vi "Dashboard Main.vi"() -> (0 "Camera Image":T3(plugin-control))   [LabVIEW 2011]
uses:
  <vilib>/Rock Robotics/WPI/Camera/WPI_CameraImageSize.ctl
  <vilib>/Rock Robotics/WPI/DriverStation/WPI_DriverStationDigitalData.ctl
  <vilib>/Utility/inputDevices.llb/keyboardAcquire.vi
  <vilib>/Utility/inputDevices.llb/closeKeyboard.vi
panel:
  out "UP":bool
  out "LEFT":bool
  out "RIGHT":bool
  out "DOWN":bool
  out "SPACE":bool
  out "X":dbl
  out "Y":dbl
  out "Target Info":T1(array[cluster])
  in  "Viewer":T2(tab)
  in  "Video Enable":bool=TRUE
  out "Processed Image":T3(plugin-control)
  in  "Range":cluster{"Lower value":sgl, "Upper value":sgl}={"Lower value"=234.67392, "Upper value"=255.0} {"Lower value" scale=0.0..255.0; "Upper value" scale=0.0..255.0}
  in  "Image Size":T4
  in  "1":bool
  in  "2":bool
  in  "3":bool
  in  "4":bool
  out "Selected Target Info":T5
  out "Buttons 1":cluster{"1":bool, "2":bool, "3":bool}
  out "Kinect 1":cluster{"X":dbl, "Y":dbl, "Z":dbl} {"X" scale=1.0..-1.0; "Y" scale=1.0..-1.0; "Z" scale=1.0..-1.0}
  out "Buttons 2":cluster{"1":bool, "2":bool, "3":bool}
  out "Kinect 2":cluster{"X":dbl, "Y":dbl, "Z":dbl} {"X" scale=1.0..-1.0; "Y" scale=1.0..-1.0; "Z" scale=1.0..-1.0}
  out "Version":string
  out "Skeleton Picture":picture
  out "Players":i8
  out "Original Image":T3(plugin-control)
  out "Latched Cordinates":i32[](array[numeric])
  out "?":i32[](array[numeric])
  out "Numeric 2":dbl
  out "Numeric":dbl
  out "distance to basket":dbl
  out "rotation angle":dbl
  in  "Basket Number":i32
  out "Dashboard Datatype Warning":string="Warning: The Dashboard Datatype used by the robot project and this dashboard do not match.\nSee diagram for more details."
  # "1"
  # "2"
  # "3"
  # "4"
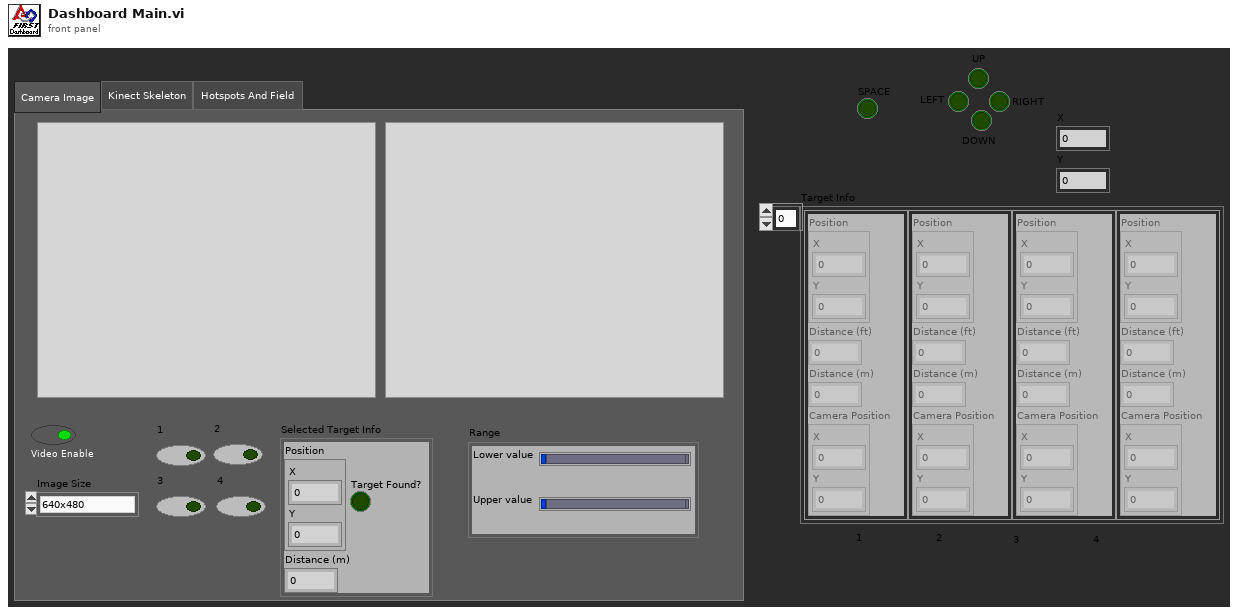
[diagram p1: front panel]
types:
  T1 = cluster{"Position":cluster{"X":dbl, "Y":dbl}, "Distance (ft)":dbl, "Distance (m)":dbl, "Camera Position":cluster{"X":dbl, "Y":dbl}}[]
  T2 = enum32{"Camera Image", "Kinect Skeleton", "Hotspots And Field "}
  T3 = typedef "IMAQ Image.ctl" = refnum<image>
  T4 = typedef "WPI_CameraImageSize.ctl" = enum16{"640x480", "320x240", "160x120"}
  T5 = cluster{"Position":cluster{"X":dbl, "Y":dbl}, "Distance (m)":dbl, "Target Found?":bool}
  T6 = typedef "Image Type" = u32
  T7 = cluster{"Coordinates[0]":i32, "Coordinates[1]":i32, "Coordinates[2]":i32, "Coordinates[3]":i32, "Coordinates[4]":i32, "Coordinates[5]":i32, "Coordinates[6]":i32, "Coordinates[7]":i32, "Coordinates[8]":i32}
  T8 = enum16{"0", "1", "2", "3", "4", "5", "6", "7", "8", "9", "A", "B", "C", "D", "E", "F", "G", "H", "I", "J", "K", "L", "M", "N", "O", "P", "Q", "R", "S", "T", "U", "V", "W", "X", "Y", "Z", "F1", "F2", "F3", "F4", "F5", "F6", "F7", "F8", "F9", "F10", "F11", "F12", "F13", "F14", "F15", "ADD", "BACK", "BACKSLASH", "CAPITAL", "COMMA", "DECIMAL", "DELETE", "DIVIDE", "DOWN", "END", "EQUALS", "ESCAPE", "GRAVE (`)", "HOME", "INSERT", "LBRACKET", "LCONTROL", "LEFT", "L ALT", "LSHIFT", "LWIN", "MINUS", "MULTIPLY", "NEXT", "NUMLOCK", "NUMPAD_0", "NUMPAD_1", "NUMPAD_2", "NUMPAD_3", "NUMPAD_4", "NUMPAD_5", "NUMPAD_6", "NUMPAD_7", "NUMPAD_8", "NUMPAD_9", "PAUSE", "PERIOD", "PRIOR (PG UP)", "RBRACKET", "RCONTROL", "RETURN", "RIGHT", "R ALT", "RSHIFT", "RWIN", "SCROLL", "SEMICOLON", "SLASH", "SPACE", "SUBTRACT", "TAB", "UP", "ENTER (num pad)", "' (quote)"}
  T9 = enum16{"0", "1", "2", "3", "4", "5", "6", "7", "8", "9", "A", "B", "C", "D", "E", "F", "G", "H", "I", "J", "K", "L", "M", "N", "O", "P", "Q", "R", "S", "T", "U", "V", "W", "X", "Y", "Z", "F1", "F2", "F3", "F4", "F5", "F6", "F7", "F8", "F9", "F10", "F11", "F12", "F13", "F14", "F15", "ADD", "BACK", "BACKSLASH", "CAPITAL", "COMMA", "DECIMAL", "DELETE", "DIVIDE", "DOWN", "END", "EQUALS", "ESCAPE", "GRAVE (`)", "HOME", "INSERT", "LBRACKET", "LCONTROL", "LEFT", "L ALT", "LSHIFT", "LWIN", "MINUS", "MULTIPLY", "NEXT", "NUMLOCK", "NUMPAD_0", "NUMPAD_1", "NUMPAD_2", "NUMPAD_3", "NUMPAD_4", "NUMPAD_5", "NUMPAD_6", "NUMPAD_7", "NUMPAD_8", "NUMPAD_9", "PAUSE", "PERIOD", "PRIOR (PG UP)", "RBRACKET", "RCONTROL", "RETURN", "RIGHT", "R ALT", "RSHIFT", "RWIN", "SCROLL", "SEMICOLON", "SLASH", "SPACE", "SUBTRACT", "TAB", "UP", "ENTER (num pad)", "' (quote)"}[]
  T10 = typedef "WPI_DriverStationDigitalData.ctl" = cluster{"Relay Fwd":u8, "Relay Rev":u8, "GPIO":u16, "GPIO_OE":u16, "PWM":cluster{"PWM[0]":u8, "PWM[1]":u8, "PWM[2]":u8, "PWM[3]":u8, "PWM[4]":u8, "PWM[5]":u8, "PWM[6]":u8, "PWM[7]":u8, "PWM[8]":u8, "PWM[9]":u8}}
  T11 = cluster{cluster{"AnalogModule[0]":cluster{"Channel[0]":sgl, "Channel[1]":sgl, "Channel[2]":sgl, "Channel[3]":sgl, "Channel[4]":sgl, "Channel[5]":sgl, "Channel[6]":sgl, "Channel[7]":sgl}, "AnalogModule[1]":cluster{"Channel[0]":sgl, "Channel[1]":sgl, "Channel[2]":sgl, "Channel[3]":sgl, "Channel[4]":sgl, "Channel[5]":sgl, "Channel[6]":sgl, "Channel[7]":sgl}}, cluster{"DigitalModule[0]":T10, "DigitalModule[1]":T10}, "Solenoid":u8}
  T12 = cluster{"Competition mode":bool, "Robot Link":bool, "Autonomous":bool, "Enabled":bool, "E-Stop":bool}
  T13 = cluster{"AnalogModule[0]":cluster{"Channel[0]":sgl, "Channel[1]":sgl, "Channel[2]":sgl, "Channel[3]":sgl, "Channel[4]":sgl, "Channel[5]":sgl, "Channel[6]":sgl, "Channel[7]":sgl}, "AnalogModule[1]":cluster{"Channel[0]":sgl, "Channel[1]":sgl, "Channel[2]":sgl, "Channel[3]":sgl, "Channel[4]":sgl, "Channel[5]":sgl, "Channel[6]":sgl, "Channel[7]":sgl}}
  T14 = cluster{"DigitalModule[0]":T10, "DigitalModule[1]":T10}
  T15 = cluster{"Channel[0]":sgl, "Channel[1]":sgl, "Channel[2]":sgl, "Channel[3]":sgl, "Channel[4]":sgl, "Channel[5]":sgl, "Channel[6]":sgl, "Channel[7]":sgl}[]
  T16 = cluster{"Channel[0]":sgl, "Channel[1]":sgl, "Channel[2]":sgl, "Channel[3]":sgl, "Channel[4]":sgl, "Channel[5]":sgl, "Channel[6]":sgl, "Channel[7]":sgl}
  T17 = typedef "LVRectTypeDef.ctl" = cluster{"left":i16, "top":i16, "right":i16, "bottom":i16}
  T18 = typedef "SkeletonTrackState.ctl" = enum32{"NotTracked", "PositionOnly", "Tracked"}
  T19 = cluster{"TrackingState":u8[], "Position":cluster{"x":sgl, "y":sgl, "z":sgl}, cluster{"x":sgl, "y":sgl, "z":sgl, sgl}[], "TrackState":T18}
  T20 = cluster{cluster{"ScaledToPercentRange":dbl, "ScaledToPercentRange":dbl, "ScaledToPercentRange":dbl}, cluster{bool, bool, bool}}[]
  T21 = typedef "LVBoundsTypeDef.ctl" = cluster{"Width":u32, "Height":u32}
  T22 = cluster{cluster{"ScaledToPercentRange":dbl, "ScaledToPercentRange":dbl, "ScaledToPercentRange":dbl}, cluster{bool, bool, bool}}
  T23 = cluster{"ScaledToPercentRange":dbl, "ScaledToPercentRange":dbl, "ScaledToPercentRange":dbl}
  T24 = cluster{"fps":i32, "compression":i32, "Image Size":T4}
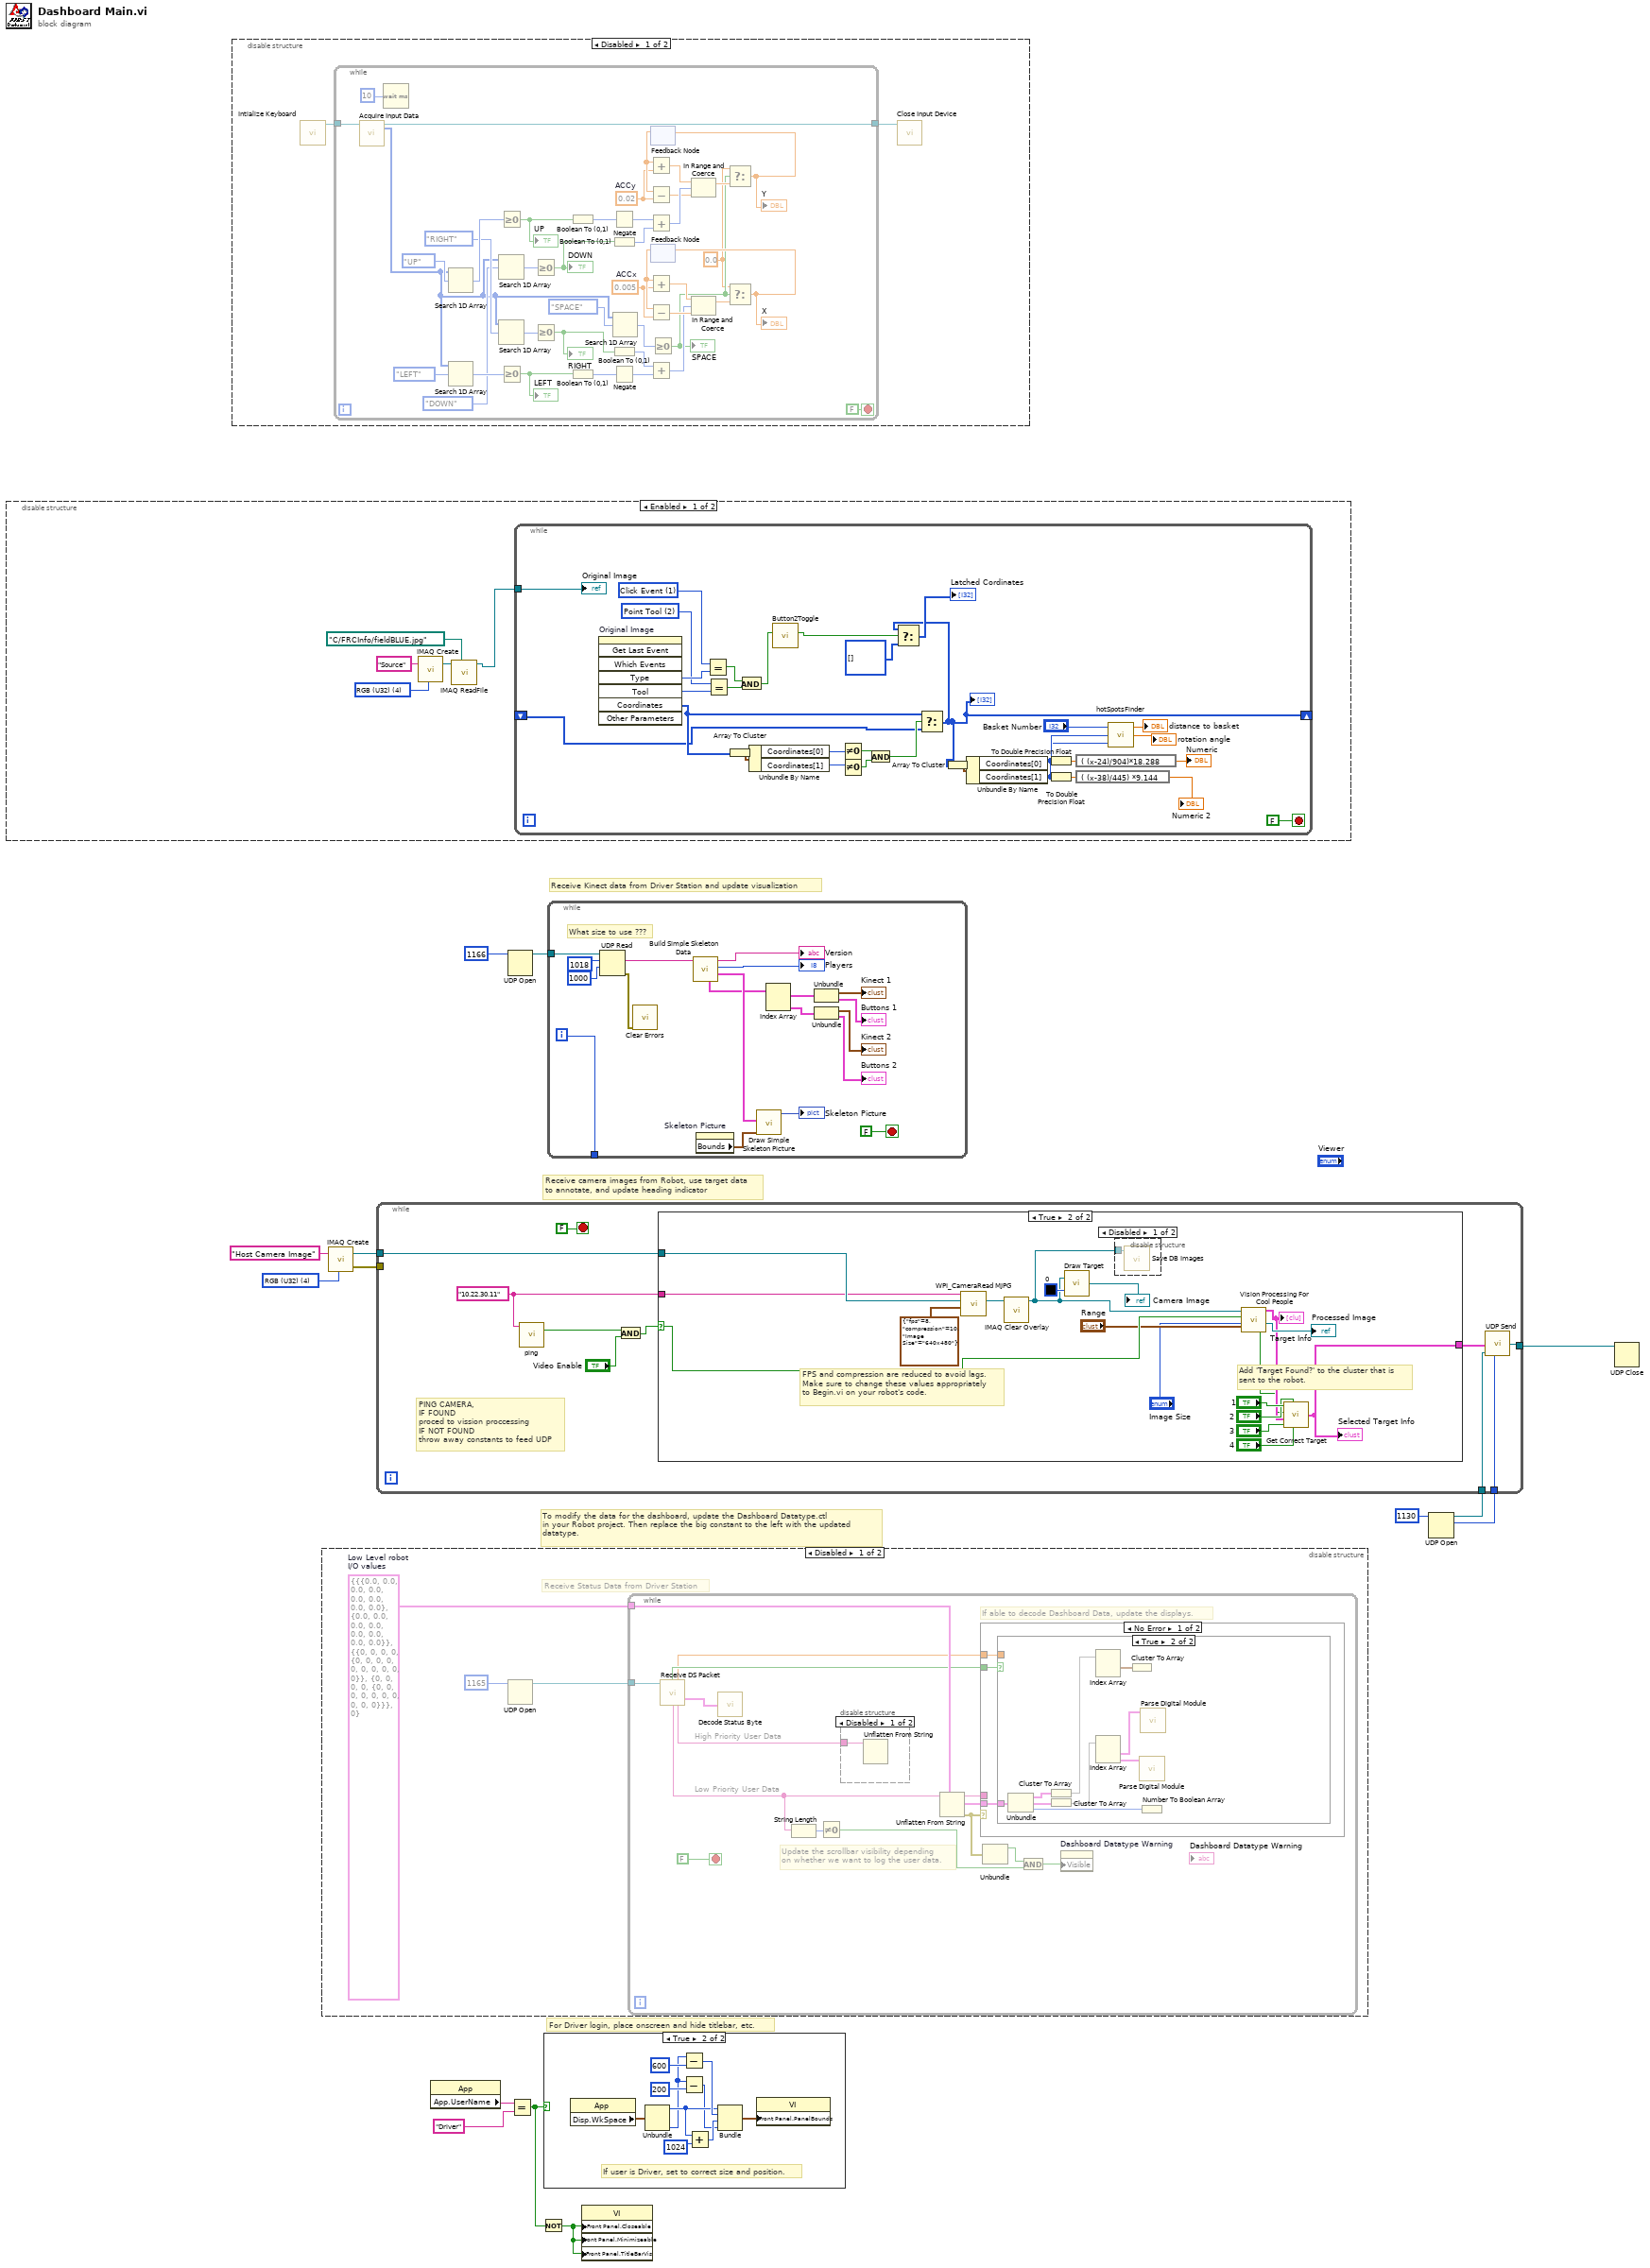
[diagram p0: block diagram]
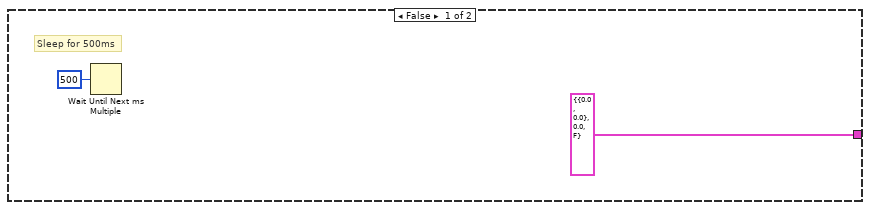
[diagram p9: hidden frame]
diagram:
  w14 = T6 4 items=["Grayscale (U8)", "Grayscale (I16)", "Grayscale (SGL)", "Complex (CSG)", "RGB (U32)", "HSL (U32)", "RGB (U64)"] ("Image Type")
  # "Receive Kinect data from Driver Station and update visualization"
  # "For Driver login, place onscreen and hide titlebar, etc."
  # "To modify the data for the dashboard, update the Dashboard Datatype.ctl\nin your Robot project. Then replace the big constant to the left with the updated\ndatatype."
  # "Receive camera images from Robot, use target data\nto annotate, and update heading indicator"
  n1 = disable-structure shown="Enabled" {
    frame Enabled {
      w15 = T6 4 items=["Grayscale (U8)", "Grayscale (I16)", "Grayscale (SGL)", "Complex (CSG)", "RGB (U32)", "HSL (U32)", "RGB (U64)", "Grayscale (U16)"] ("Image Type")
      n2 = call "IMAQ Create"("Image Name"="Source", "Image Type"=w15) -> ("New Image"=w17:T3)  [unwired: 2 in, 2 out]
      n3 = call "IMAQ ReadFile"("File Path"=path "C:/FRCInfo/fieldBLUE.jpg", "Image"=w17) -> ("Image Out"=w16:T3)  [unwired: 5 in, 4 out]
      n4 = while {
        tunnel: w16 -> [w44]
        shift-right: [w29] -> _
        shift-left: _ -> [w34]
        stop <- FALSE stop-if-true
        w45 = 2 items=["None", "Selection Tool", "Point Tool", "Line Tool", "Rectangle Tool", "Oval Tool", "Polygon Tool", "ClosedFreehandTool", "Annulus Tool", "Rotated Rectangle Tool", "Zoom Tool", "Pan Tool", "Polyline Tool", "Freehand Tool"] ("Tool")
        w46 = 1 items=["No Event"=0, "Click Event"=1, "Draw Event"=2, "Size Event"=4, "Scroll Event"=5, "Double Click Event"=8] ("Type")
        n5 = invoke on="Original Image" class="ImageControl" method="Get Last Event"() -> ("Type"=w47:i32, "Tool"=w50:i32, "Coordinates"=w35:i32[])  [unwired: 8 in, 5 out]
        n6 = Equal?(x=w46, y=w47) -> (x = y?=w48:bool)
        n7 = Equal?(x=w45, y=w50) -> (x = y?=w49:bool)
        n8 = Array To Cluster(array=w35) -> (cluster=w41:T7)
        n9 = And(x=w48, y=w49) -> (x .and. y?=w42:bool)
        n10 = Unbundle By Name(w41) -> ("Coordinates[0]"=w39:i32, "Coordinates[1]"=w37:i32)
        n11 = call "Button2Toggle.vi"("Boolean"=w42) -> ("Latched Boolean"=w33:bool)  [unwired: 9 in, 1 out]
        n12 = Not Equal To 0?(x=w37) -> (x != 0?=w38:bool)
        n13 = Not Equal To 0?(x=w39) -> (x != 0?=w40:bool)
        n14 = And(x=w40, y=w38) -> (x .and. y?=w36:bool)
        n15 = Select(t=w35, s=w36, f=w34) -> (s? t:f=w29:i32[])
        "?" <- w29
        n16 = Select(t=w29, s=w33, f=i32[] [] ("Coordinates")) -> (s? t:f=→"Latched Cordinates":i32[])
        n17 = Array To Cluster(array=w29) -> (cluster=w30:T7)
        n18 = Unbundle By Name(w30) -> ("Coordinates[0]"=w24:i32, "Coordinates[1]"=w23:i32)
        n19 = To Double Precision Float(number=w24) -> (double precision float=w27:dbl)
        n20 = To Double Precision Float(number=w23) -> (double precision float=w28:dbl)
        n21 = expression code="( (x-24)/904)*18.288"(w27) -> (→"Numeric":dbl)
        n22 = expression code="( (x-38)/445) *9.144"(w28) -> (→"Numeric 2":dbl)
        n23 = call "hotSpotsFinder.vi"("y"=w23, "x"=w24, "Basket Number"="Basket Number") -> ("rotation angle"=→"rotation angle":dbl, "distance to basket"=→"distance to basket":dbl)  [unwired: 1 out]
        "Original Image" <- w44
      }
    }
    frame Disabled {
    }
  }
  n24 = disable-structure shown="Disabled" {
    frame Disabled {
      n25 = call <vilib>:"Intialize Keyboard.vi"() -> ("device ID"=w52:refnum<k1>)  [unwired: 1 in, 10 out]
      n26 = while {
        tunnel: [w92] -> w51
        tunnel: w52 -> [w91]
        stop <- FALSE stop-if-true
        w54 = 0.005  # ACCx
        w55 = 0.0 ("t")
        w61 = 0.02  # ACCy
        n27 = call-poly <vilib>:"Acquire Input Data.vi"("device ID"=w91) -> ("device ID"=w92:refnum<k1>, "keys pressed"=w82:T9)  [unwired: 1 in, 16 out]
        n28 = Wait (ms)(milliseconds to wait=u32 10) -> ()  [unwired: 1 out]
        n29 = Search 1D Array(1D array=w82, element=T8."UP" ("keys pressed[0]")) -> (index of element=w89:i32)  [unwired: 1 in]
        n30 = Search 1D Array(1D array=w82, element=T8."LEFT" ("keys pressed[0]")) -> (index of element=w88:i32)  [unwired: 1 in]
        n31 = Greater Or Equal To 0?(x=w89) -> (x >= 0?=w79:bool)
        "UP" <- w79
        n32 = Search 1D Array(1D array=w82, element=T8."DOWN" ("keys pressed[0]")) -> (index of element=w86:i32)  [unwired: 1 in]
        n33 = Search 1D Array(1D array=w82, element=T8."RIGHT" ("keys pressed[0]")) -> (index of element=w87:i32)  [unwired: 1 in]
        n34 = Greater Or Equal To 0?(x=w88) -> (x >= 0?=w78:bool)
        "LEFT" <- w78
        n35 = Greater Or Equal To 0?(x=w86) -> (x >= 0?=w76:bool)
        "DOWN" <- w76
        n36 = Greater Or Equal To 0?(x=w87) -> (x >= 0?=w77:bool)
        "RIGHT" <- w77
        n37 = Boolean To (0,1)(Boolean=w79) -> (0, 1=w75:i16)
        n38 = Boolean To (0,1)(Boolean=w78) -> (0, 1=w71:i16)
        n39 = Negate(x=w75) -> (-x=w74:i16)
        n40 = Boolean To (0,1)(Boolean=w76) -> (0, 1=w73:i16)
        n41 = Boolean To (0,1)(Boolean=w77) -> (0, 1=w72:i16)
        n42 = Negate(x=w71) -> (-x=w70:i16)
        n43 = Search 1D Array(1D array=w82, element=T8."SPACE" ("keys pressed[0]")) -> (index of element=w80:i32)  [unwired: 1 in]
        n44 = Add(x=w74, y=w73) -> (x+y=w69:i16)
        n45 = Add(x=w72, y=w70) -> (x+y=w62:i16)
        n46 = feedback #1() -> (w68:dbl)  [unwired: 1 in]
        n47 = Add(x=w68, y=w61) -> (x+y=w67:dbl)
        n48 = Subtract(x=w68, y=w61) -> (x-y=w66:dbl)
        n49 = feedback #2() -> (w63:dbl)  [unwired: 1 in]
        n50 = Add(x=w63, y=w54) -> (x+y=w64:dbl)
        n51 = Subtract(x=w63, y=w54) -> (x-y=w65:dbl)
        n52 = Greater Or Equal To 0?(x=w80) -> (x >= 0?=w56:bool)
        "SPACE" <- w56
        n53 = In Range and Coerce(upper limit=w67, x=w69, lower limit=w66) -> (coerced(x)=w57:dbl)  [unwired: 1 out]
        n54 = In Range and Coerce(upper limit=w64, x=w62, lower limit=w65) -> (coerced(x)=w60:dbl)  [unwired: 1 out]
        n55 = Select(t=w55, s=w56, f=w57) -> (s? t:f=w58:dbl)
        "Y" <- w58
        n56 = feedback-in #1(w58) -> ()
        n57 = Select(t=w55, s=w56, f=w60) -> (s? t:f=w59:dbl)
        "X" <- w59
        n58 = feedback-in #2(w59) -> ()
      }
      n59 = call-poly <vilib>:"Close Input Device.vi"("device ID"=w51) -> ()  [unwired: 1 in, 9 out]
    }
    frame Enabled {
    }
  }
  n60 = disable-structure shown="Disabled" {
    frame Disabled {
      w94 = T11 {{"AnalogModule[0]"={"Channel[0]"=0.0, "Channel[1]"=0.0, "Channel[2]"=0.0, "Channel[3]"=0.0, "Channel[4]"=0.0, "Channel[5]"=0.0, "Channel[6]"=0.0, "Channel[7]"=0.0}, "AnalogModule[1]"={"Channel[0]"=0.0, "Channel[1]"=0.0, "Channel[2]"=0.0, "Channel[3]"=0.0, "Channel[4]"=0.0, "Channel[5]"=0.0, "Channel[6]"=0.0, "Channel[7]"=0.0}}, {"DigitalModule[0]"={"Relay Fwd"=0, "Relay Rev"=0, "GPIO"=0, "GPIO_OE"=0, "PWM"={"PWM[0]"=0, "PWM[1]"=0, "PWM[2]"=0, "PWM[3]"=0, "PWM[4]"=0, "PWM[5]"=0, "PWM[6]"=0, "PWM[7]"=0, "PWM[8]"=0, "PWM[9]"=0}}, "DigitalModule[1]"={"Relay Fwd"=0, "Relay Rev"=0, "GPIO"=0, "GPIO_OE"=0, "PWM"={"PWM[0]"=0, "PWM[1]"=0, "PWM[2]"=0, "PWM[3]"=0, "PWM[4]"=0, "PWM[5]"=0, "PWM[6]"=0, "PWM[7]"=0, "PWM[8]"=0, "PWM[9]"=0}}}, "Solenoid"=0}  # Low Level robot I/O values
      # "Receive Status Data from Driver Station"
      n61 = UDP Open(11:u16 1165 ("port")) -> (port=w95:refnum<k16>)  [unwired: 2 in, 4 out]
      n62 = while {
        tunnel: w95 -> [w109]
        tunnel: w94 -> [w108]
        stop <- FALSE stop-if-true
        # "High Priority User Data"
        # "Low Priority User Data"
        # "Update the scrollbar visibility depending\non whether we want to log the user data."
        # "If able to decode Dashboard Data, update the displays."
        n63 = call "Receive DS Packet.vi"("Recv Socket"=w109) -> ("New Dashboard Data"=w105:bool, "Battery"=w97:sgl, "Status"=w110:T12, "Low Priority User Data"=w99:string, "High Priority User Data"=w98:string)  [unwired: 1 in, 9 out]
        n64 = call "Decode Status Byte.vi"("Status Byte"=w110) -> ()  [unwired: 2 out]
        n65 = String Length(string=w99) -> (length=w100:i32)
        n66 = Not Equal To 0?(x=w100) -> (x != 0?=w103:bool)
        n67 = disable-structure shown="Disabled" {
          disable-tunnel: w98 -> [w112 _]
          frame Disabled {
            n68 = Unflatten From String(binary string=w112) -> ()  [unwired: 2 in, 5 out]
          }
          frame Enabled {
          }
        }
        n69 = Unflatten From String(type=w108, binary string=w99) -> (rest of the binary string=w101:string, value=w107:T11, error out=w106:errorcluster)  [unwired: 1 in, 2 out]
        n70 = case shown="No Error" w106 {
          tunnel: w107 -> [w115 _]
          tunnel: w105 -> [w114 _]
          tunnel: w101 -> [_ _]
          tunnel: w97 -> [w113 _]
          frame No Error {
            n71 = case shown="True" w114 {
              tunnel: w115 -> [_ w120]
              tunnel: w113 -> [_ _]
              frame False {
                # "Don't update if the robot hasn't sent new data"
              }
              frame True {
                n72 = Unbundle(w120) -> (w117:T13, w118:T14, "Solenoid"=w119:u8)
                n73 = Cluster To Array(cluster=w117) -> (array=w124:T15)
                n74 = Cluster To Array(cluster=w118) -> (array=w123:T10[])
                n75 = Index Array(array=w124) -> (element #1=w116:T16)  [unwired: 2 in, 1 out]
                n76 = Index Array(array=w123) -> (element #1=w122:T10, element #2=w121:T10)  [unwired: 2 in]
                n77 = Cluster To Array(cluster=w116) -> ()  [unwired: 1 out]
                n78 = call "Parse Digital Module.vi"("DigitalModule"=w121) -> ()  [unwired: 11 out]
                n79 = Number To Boolean Array(number=w119) -> ()  [unwired: 1 out]
                n80 = call "Parse Digital Module.vi"("DigitalModule"=w122) -> ()  [unwired: 11 out]
              }
            }
          }
          frame Error {
            # "Your datatypes don't match. The Dashboard Datatype.ctl in your Robot project\nand the big constant to the left of the loop need to match."
          }
        }
        n81 = Unbundle(w106) -> ("status"=w102:bool)  [unwired: 2 out]
        n82 = And(x=w102, y=w103) -> (x .and. y?=w104:bool)
        n83 = property on="Dashboard Datatype Warning" class="Str"("Visible"=w104) -> ()  [unwired: 2 in, 2 out]
      }
    }
    frame Enabled {
    }
  }
  n84 = call "IMAQ Create"("Image Name"="Host Camera Image", "Image Type"=w14) -> ("New Image"=w12:T3, "error out"=w11:errorcluster)  [unwired: 2 in, 1 out]
  n85 = property class="App"() -> ("App.UserName"=w9:string)  [unwired: 2 in, 2 out]
  n86 = UDP Open(11:u16 1166 ("port")) -> (port=w5:refnum<k16>)  [unwired: 2 in, 4 out]
  n87 = Equal?(x=w9, y="Driver") -> (x = y?=w8:bool)
  n88 = Not(x=w8) -> (.not. x?=w7:bool)
  n89 = case shown="True" w8 {
    frame False {
    }
    frame True {
      # "If user is Driver, set to correct size and position."
      n90 = property class="App"() -> ("Disp.WkSpace"=w134:T17)  [unwired: 2 in, 2 out]
      n91 = Unbundle(w134) -> ("left"=w129:i16, "bottom"=w125:i16)  [unwired: 2 out]
      n92 = Subtract(x=w125, y=600) -> (x-y=w131:i32)
      n93 = Subtract(x=w125, y=200) -> (x-y=w126:i32)
      n94 = Add(x=w129, y=1024) -> (x+y=w130:i32)
      n95 = Bundle("left"=w129, w131, w130, w126) -> (w133:cluster{"left":i16, i32, i32, i32})  [unwired: 1 out]
      n96 = property class="VI"("Front Panel.PanelBounds"=w133) -> ()  [unwired: 2 in, 2 out]
    }
  }
  n97 = while {
    tunnel: w5 -> [w151]
    tunnel: [w135] -> _
    i -> [w135]
    stop <- FALSE stop-if-true
    # "What size to use ???"
    n98 = UDP Read(connection ID=w151, max size (548)=1018 ("bytes to read"), timeout ms (25000)=1000) -> (data out=w145:string, error out=w143:errorcluster)  [unwired: 1 in, 3 out]
    n99 = call <vilib>:"Clear Errors.vi"("error in (no error)"=w143) -> ()  [unwired: 6 in, 1 out]
    n100 = call "Build Simple Skeleton Data.vi"("data out"=w145) -> ("Skeleton Data"=w146:T19, "NumPlayers"=→"Players":i8, "Version String"=→"Version":string, "Simple Joystick Info"=w142:T20)  [unwired: 6 in, 1 out]
    n101 = property on="Skeleton Picture" class="Pict"() -> ("Bounds"=w147:T21)  [unwired: 2 in, 2 out]
    n102 = call "Draw Simple Skeleton Picture.vi"("Bounds"=w147, "Simple Skeleton"=w146) -> ("new picture out"=→"Skeleton Picture":picture)  [unwired: 9 in]
    n103 = Index Array(array=w142) -> (element #1=w141:T22, element #2=w140:T22)  [unwired: 2 in]
    n104 = Unbundle(w141) -> (→"Kinect 1":T23, →"Buttons 1":cluster{bool, bool, bool})
    n105 = Unbundle(w140) -> (→"Kinect 2":T23, →"Buttons 2":cluster{bool, bool, bool})
  }
  n106 = property class="VI"("Front Panel.Closeable"=w7, "Front Panel.Minimizeable"=w7, "Front Panel.TitleBarVis"=w7) -> ()  [unwired: 2 in, 2 out]
  n107 = UDP Open(11:u16 1130 ("port")) -> (port=w3:refnum<k16>, 2:w2:u16)  [unwired: 1 in, 4 out]
  n108 = while {
    tunnel: w12 -> [w162]
    tunnel: w11 -> [_]
    tunnel: w3 -> [w161]
    tunnel: w2 -> [w160]
    tunnel: [w159] -> w1
    stop <- FALSE stop-if-true
    w157 = "10.22.30.11" ("address")
    # "PING CAMERA,\nIF FOUND \nproced to vission proccessing \nIF NOT FOUND\nthrow away constants to feed UDP"
    n109 = call "ping.vi"("host"=w157) -> ("found?"=w155:bool)  [unwired: 8 in, 2 out]
    n110 = And(x=w155, y="Video Enable") -> (x .and. y?=w156:bool)
    n111 = case shown="True" w156 {
      selector: w156 -> [_ w182]
      tunnel: w162 -> [_ w183]
      tunnel: [T5 {"Position"={"X"=0.0, "Y"=0.0}, "Distance (m)"=0.0, "Target Found?"=FALSE} ("Selected Target Info") w181] -> w158
      tunnel: w157 -> [_ w180]
      frame False {
        # "Sleep for 500ms"
        n112 = Wait Until Next ms Multiple(millisecond multiple=u32 500) -> ()  [unwired: 1 out]
      }
      frame True {
        # "Add 'Target Found?' to the cluster that is\nsent to the robot."
        # "FPS and compression are reduced to avoid lags.\nMake sure to change these values appropriately\nto Begin.vi on your robot's code."
        n113 = call <vilib>:"WPI_CameraRead MJPG.vi"("Camera Settings"=T24 {"fps"=8, "compression"=10, "Image Size"=enum."640x480"}, "Image"=w183, "address"=w180) -> ("Image Out"=w179:T3)  [unwired: 7 in, 1 out]
        n114 = call "IMAQ Clear Overlay"("Image"=w179) -> ("Image Out"=w167:T3)  [unwired: 2 in, 8 out]
        n115 = call "Draw Target.vi"("Color"=u32 0, "Original Image"=w167) -> ("Image Out"=→"Camera Image":T3)
        n116 = disable-structure shown="Disabled" {
          disable-tunnel: w167 -> [w184 _]
          frame Disabled {
            n117 = call "Save DB Images.vi"("Image"=w184) -> ()  [unwired: 2 in, 1 out]
          }
          frame Enabled {
          }
        }
        n118 = call "Vision Processing For Cool People.vi"("Range"="Range", "Image Size"="Image Size", "View 2"=w182, "Original Image"=w167) -> ("Target Found?"=w166:bool, "Processed Image"=→"Processed Image":T3, "Target Info"=w170:T1)  [unwired: 1 out]
        "Target Info" <- w170
        n119 = call "Get Correct Target.vi"("4"="4", "2"="2", "3"="3", "Target Info"=w170, "Target Found?"=w166, "1"="1") -> ("Selected Target Info"=w181:T5)
        "Selected Target Info" <- w181
      }
    }
    n120 = call "UDP Send.vi"("Selected Target Info"=w158, "connection ID"=w161, "port"=w160) -> ("connection ID out"=w159:refnum<k16>)  [unwired: 2 in]
  }
  n121 = UDP Close(connection ID=w1) -> ()  [unwired: 1 in, 2 out]
